vi "FTDI_MPSSE_Ini.vi"(8 "error in (no error)":errorcluster, 10 "Channel Nmb":u8) -> (0 "error out":errorcluster, 1 "Serial number":string, 2 "Ini Status":bool, 3 "Handler":u32, 5 "Description":string)   [LabVIEW 2018]
uses:
  dll/libMPSSE.dll
  PROJEKT/NIKO/Labview/Niko V6_A/FTDI SPI/libMPSSE-SPI.lvlib
panel:
  out "Flags":u32 format="%b"
  out "Type":u32
  out "ID":u32 format="%08x"
  out "LocId":u32
  out "ftHandle":u32 format="%08x"
  out "numChannels":i32
  # "FTDI Info"
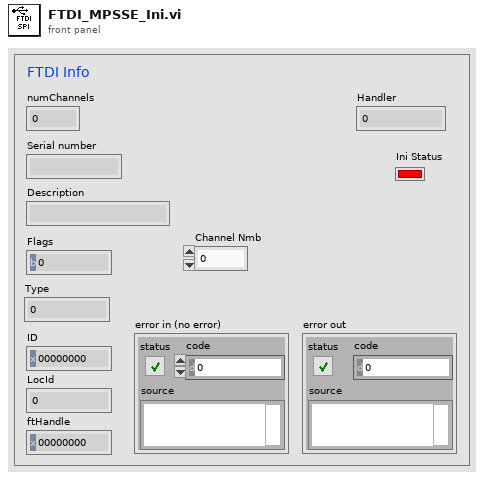
[diagram p1: front panel]
types:
  T1 = cluster{"Flags":u32, "Type":u32, "ID":u32, "LocId":u32, "SerialNumber[0]":i8, "SerialNumber[1]":i8, "SerialNumber[2]":i8, "SerialNumber[3]":i8, "SerialNumber[4]":i8, "SerialNumber[5]":i8, "SerialNumber[6]":i8, "SerialNumber[7]":i8, "SerialNumber[8]":i8, "SerialNumber[9]":i8, "SerialNumber[10]":i8, "SerialNumber[11]":i8, "SerialNumber[12]":i8, "SerialNumber[13]":i8, "SerialNumber[14]":i8, "SerialNumber[15]":i8, "Description[0]":i8, "Description[1]":i8, "Description[2]":i8, "Description[3]":i8, "Description[4]":i8, "Description[5]":i8, "Description[6]":i8, "Description[7]":i8, "Description[8]":i8, "Description[9]":i8, "Description[10]":i8, "Description[11]":i8, "Description[12]":i8, "Description[13]":i8, "Description[14]":i8, "Description[15]":i8, "Description[16]":i8, "Description[17]":i8, "Description[18]":i8, "Description[19]":i8, "Description[20]":i8, "Description[21]":i8, "Description[22]":i8, "Description[23]":i8, "Description[24]":i8, "Description[25]":i8, "Description[26]":i8, "Description[27]":i8, "Description[28]":i8, "Description[29]":i8, "Description[30]":i8, "Description[31]":i8, "Description[32]":i8, "Description[33]":i8, "Description[34]":i8, "Description[35]":i8, "Description[36]":i8, "Description[37]":i8, "Description[38]":i8, "Description[39]":i8, "Description[40]":i8, "Description[41]":i8, "Description[42]":i8, "Description[43]":i8, "Description[44]":i8, "Description[45]":i8, "Description[46]":i8, "Description[47]":i8, "Description[48]":i8, "Description[49]":i8, "Description[50]":i8, "Description[51]":i8, "Description[52]":i8, "Description[53]":i8, "Description[54]":i8, "Description[55]":i8, "Description[56]":i8, "Description[57]":i8, "Description[58]":i8, "Description[59]":i8, "Description[60]":i8, "Description[61]":i8, "Description[62]":i8, "Description[63]":i8, "ftHandle":u32}
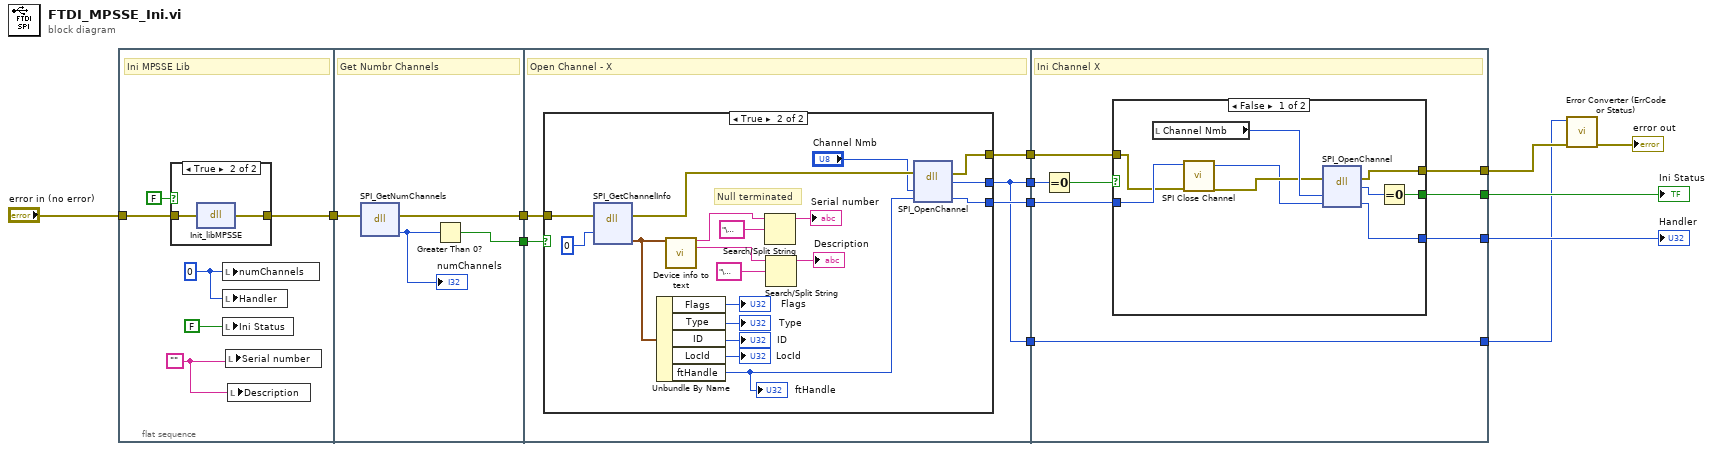
[diagram p0: block diagram]
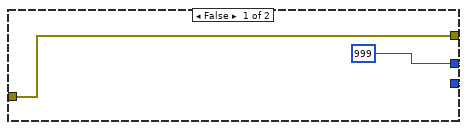
[diagram p3: hidden frame]
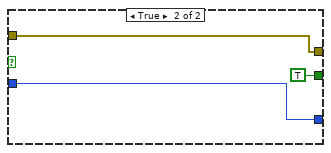
[diagram p4: hidden frame]
diagram:
  n1 = flat-sequence {
    tunnel: [w19] -> w13
    tunnel: "error in (no error)" -> [w15]
    tunnel: w13 -> [w26]
    tunnel: [w25] -> w12
    tunnel: [w23] -> w11
    tunnel: w12 -> [w31]
    tunnel: w11 -> [w30]
    tunnel: [w27] -> w10
    tunnel: [w29] -> w9
    tunnel: [w28] -> w8
    tunnel: [w27] -> w2
    tunnel: w10 -> [w60]
    tunnel: w9 -> [w59]
    tunnel: w8 -> [w58]
    tunnel: [w57] -> w6
    tunnel: [w56] -> w7
    tunnel: [w55] -> w4
    tunnel: [w54] -> w3
    tunnel: w2 -> [w54]
    frame #0 {
      w16 = ""
      w18 = 0 ("numChannels")
      # "Ini MPSSE Lib"
      n2 = case shown="True" FALSE {
        tunnel: [w20 w22] -> w19
        tunnel: w15 -> [w20 w21]
        frame False {
        }
        frame True {
          n3 = dll-call lib="D:/LABVIEW/SEQUENSER_SNA/Ver_12/FTDI SPI/dll/libMPSSE.dll" fn="Init_libMPSSE"(error in=w21) -> (error out=w22:errorcluster)  [unwired: 3 in, 1 out]
        }
      }
      n4 = local write "numChannels"(w18) -> ()
      n5 = local write "Handler"(w18) -> ()
      n6 = local write "Ini Status"(FALSE ("Ini Status")) -> ()
      n7 = local write "Serial number"(w16) -> ()
      n8 = local write "Description"(w16) -> ()
    }
    frame #1 {
      # "Get Numbr Channels"
      n9 = dll-call lib="D:/LABVIEW/SEQUENSER_SNA/Ver_12/FTDI SPI/dll/libMPSSE.dll" fn="SPI_GetNumChannels"(error in=w26) -> (error out=w25:errorcluster, "numChannels"=w24:i32)  [unwired: 4 in, 1 out]
      "numChannels" <- w24
      n10 = Greater Than 0?(x=w24) -> (x > 0?=w23:bool)
    }
    frame #2 {
      # "Open Channel - X"
      n11 = case shown="True" w30 {
        tunnel: w31 -> [w32 w47]
        tunnel: [w33 w44] -> w27
        tunnel: [w33 w43] -> w28
        tunnel: [w32 w42] -> w29
        frame False {
          w33 = u32 999 ("return type")
        }
        frame True {
          # "Null terminated"
          n12 = dll-call lib="D:/LABVIEW/SEQUENSER_SNA/Ver_12/FTDI SPI/dll/libMPSSE.dll" fn="SPI_GetChannelInfo"(error in=w47, "index"=0) -> (error out=w45:errorcluster, "chanInfo out"=w52:T1)  [unwired: 5 in, 1 out]
          n13 = Unbundle By Name(w52) -> ("Flags"=→"Flags":u32, "Type"=→"Type":u32, "ID"=→"ID":u32, "LocId"=→"LocId":u32, "ftHandle"=w35:u32)
          "ftHandle" <- w35
          n14 = call "Device info to text.vi"("chanInfo out"=w52) -> ("Serial number"=w49:string, "Description"=w48:string)  [unwired: 13 in]
          n15 = Search/Split String(string=w49, search string/char (-)="\u0000") -> (substring before match=→"Serial number":string)  [unwired: 1 in, 2 out]
          n16 = Search/Split String(string=w48, search string/char (-)="\u0000") -> (substring before match=→"Description":string)  [unwired: 1 in, 2 out]
          n17 = dll-call lib="D:/LABVIEW/SEQUENSER_SNA/Ver_12/FTDI SPI/dll/libMPSSE.dll" fn="SPI_OpenChannel"(error in=w45, "index"="Channel Nmb", "handle"=w35) -> (error out=w42:errorcluster, "return type"=w44:u32, "handle"=w43:u32)  [unwired: 3 in, 1 out]
        }
      }
    }
    frame #3 {
      # "Ini Channel X"
      n18 = Equal To 0?(x=w60) -> (x = 0?=w53:bool)
      n19 = case shown="False" w53 {
        tunnel: w58 -> [w64 w71]
        tunnel: w59 -> [w63 w70]
        tunnel: [w69 TRUE] -> w56
        tunnel: [w65 w71] -> w57
        tunnel: [w67 w70] -> w55
        frame False {
          n20 = local read "Channel Nmb"() -> (w66:u8)
          n21 = call "SPI Close Channel.vi"("error in (no error)"=w63, "handle"=w64) -> ("error out"=w62:errorcluster, "handle out"=w61:u32)  [unwired: 7 in, 1 out]
          n22 = dll-call lib="D:/LABVIEW/SEQUENSER_SNA/Ver_12/FTDI SPI/dll/libMPSSE.dll" fn="SPI_OpenChannel"(error in=w62, "index"=w66, "handle"=w61) -> (error out=w67:errorcluster, "return type"=w68:u32, "handle"=w65:u32)  [unwired: 3 in, 1 out]
          n23 = Equal To 0?(x=w68) -> (x = 0?=w69:bool)
        }
        frame True {
        }
      }
    }
  }
  n24 = call "Error Converter (ErrCode or Status).vi"("error in (no error)"=w4, "error code"=w3) -> ("error out"=→"error out":errorcluster)  [unwired: 9 in]
  "Handler" <- w6
  "Ini Status" <- w7
